vi "Helper SubVI - TDR Signal Simulation.vi"(6 "test parameters":T2={"Sample Rate [Hz]"=1000000.0, "Max Thickness [m]"=1.0, "SNR [dB]"=20.0} {"SNR [dB]" format="%.2f"; "Max Thickness [m]" format="%.2f"; "Sample Rate [Hz]" format="%.2p"}, 9 "target parameters":T1={"Reflectance"=0.0, "Phase Shift [Deg]"=-63.20559286450312} {"Reflectance" format="%.2f"}, 10 "path parameters":T3={"Thickness [m]"=0.43125, "Attenuation [dB/m]"=20.0, "Sonic Speed [m/s]"=1500.0} {"Sonic Speed [m/s]" format="%.2p"; "Attenuation [dB/m]" format="%.2f"; "Thickness [m]" format="%.4f"}, 11 "source chirplet":T4={"F Central [Hz]"=50000.0, "Bandwidth [Hz]"=50000.0, "Chirplet Length [m]"=0.2, "Amplitude [EU]"=10.0} {"Amplitude [EU]" format="%.2f"; "F Central [Hz]" format="%.2p"; "Bandwidth [Hz]" format="%.2p"; "Chirplet Length [m]" format="%.4f"}) -> (1 "noise":dbl=0.01 format="%.0p", 2 "incident chirplet":T5={"alpha"=0.00275625, "t0"=133.33333333333334, "omega"=0.314, "beta"=0.004710000000000001} {"beta" step=0.0001 format="%.2e"; "omega" format="%.2e"; "t0" format="%.3e"; "alpha" format="%.2e"}, 3 "time waveform":waveform(dbl), 4 "thickness between 2 samples":dbl format="%.2e")   [LabVIEW 2023]
doc: "Simulates a Time Domain Reflectometry (TDR) signal, which contains both the transmitted and the reflected chirplets."
uses:
  <vilib>/Analysis/NI_AALBase.lvlib
panel:
  out "length [sample]":i32=1600
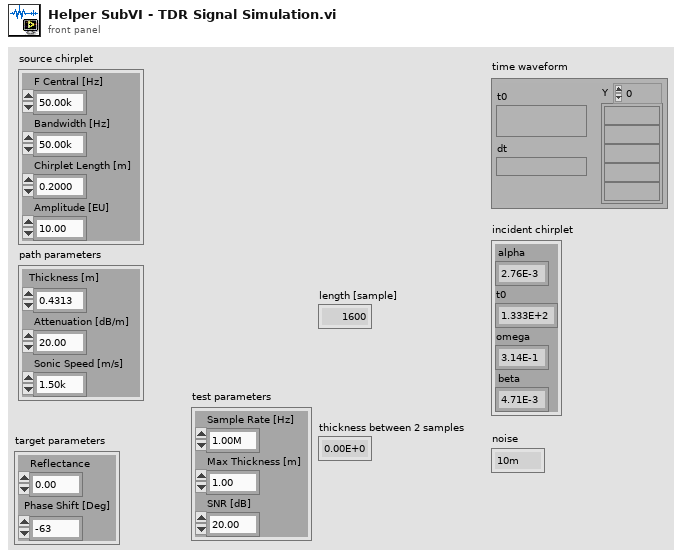
[diagram p1: front panel]
types:
  T1 = cluster{"Reflectance":dbl, "Phase Shift [Deg]":dbl}
  T2 = cluster{"Sample Rate [Hz]":dbl, "Max Thickness [m]":dbl, "SNR [dB]":dbl}
  T3 = cluster{"Thickness [m]":dbl, "Attenuation [dB/m]":dbl, "Sonic Speed [m/s]":dbl}
  T4 = cluster{"F Central [Hz]":dbl, "Bandwidth [Hz]":dbl, "Chirplet Length [m]":dbl, "Amplitude [EU]":dbl}
  T5 = cluster{"alpha":dbl, "t0":dbl, "omega":dbl, "beta":dbl}
  T6 = cluster{"F Central [Hz]":dbl, "Bandwidth [Hz]":dbl, "Chirplet Length [m]":dbl}
  T7 = cluster{"Sample Rate [Hz]":dbl, "Sonic Speed [m/s]":dbl}
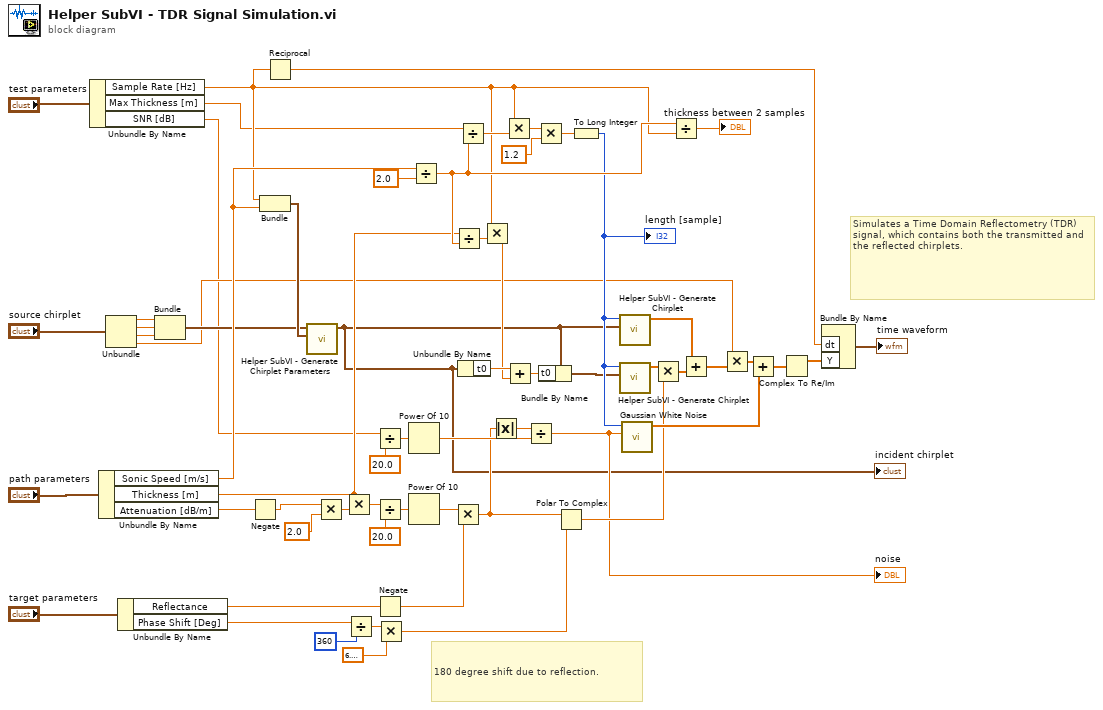
[diagram p0: block diagram]
diagram:
  # "Simulates a Time Domain Reflectometry (TDR) signal, which contains both the transmitted and the reflected chirplets."
  # "180 degree shift due to reflection."
  n1 = Unbundle By Name("test parameters") -> ("Sample Rate [Hz]"=w28:dbl, "Max Thickness [m]"=w27:dbl, "SNR [dB]"=w13:dbl)
  n2 = Unbundle By Name("path parameters") -> ("Sonic Speed [m/s]"=w30:dbl, "Thickness [m]"=w31:dbl, "Attenuation [dB/m]"=w32:dbl)
  n3 = Unbundle("source chirplet") -> ("F Central [Hz]"=w25:dbl, "Bandwidth [Hz]"=w24:dbl, "Chirplet Length [m]"=w23:dbl, "Amplitude [EU]"=w21:dbl)
  n4 = Unbundle By Name("target parameters") -> ("Reflectance"=w18:dbl, "Phase Shift [Deg]"=w19:dbl)
  n5 = Bundle("F Central [Hz]"=w25, "Bandwidth [Hz]"=w24, "Chirplet Length [m]"=w23) -> (w22:T6)  [unwired: 1 out]
  n6 = Negate(x=w32) -> (-x=w4:dbl)
  n7 = Bundle("Sample Rate [Hz]"=w28, "Sonic Speed [m/s]"=w30) -> (w36:T7)  [unwired: 1 out]
  n8 = Reciprocal(x=w28) -> (1/x=w8:dbl)
  n9 = call "Helper SubVI - Generate Chirplet Parameters.vi"("test conditions"=w36, "chirplet settings"=w22) -> ("chirplet parameters"=w2:T5)  [unwired: 1 in, 8 out]
  "incident chirplet" <- w2
  n10 = Multiply(x=w4, y=2.0) -> (x*y=w5:dbl)
  n11 = Multiply(x=w31, y=w5) -> (x*y=w51:dbl)
  n12 = Divide(x=w19, y=360) -> (x/y=w38:dbl)
  n13 = Divide(x=w13, y=20.0) -> (x/y=w12:dbl)
  n14 = Divide(x=w51, y=20.0) -> (x/y=w49:dbl)
  n15 = Negate ("180 degree shift due to reflection")(x=w18) -> (-x=w16:dbl)
  n16 = Multiply(x=w38, y=6.283185307179586 ("Pi Multiplied By 2")) -> (x*y=w15:dbl)
  n17 = Power Of 10(x=w12) -> (10^x=w11:dbl)
  n18 = Power Of 10(x=w49) -> (10^x=w47:dbl)
  n19 = Divide(x=w30, y=2.0) -> (x/y=w41:dbl)
  n20 = Multiply(x=w47, y=w16) -> (x*y=w10:dbl)
  n21 = Divide(x=w31, y=w41) -> (x/y=w55:dbl)
  n22 = Divide(x=w27, y=w41) -> (x/y=w56:dbl)
  n23 = Unbundle By Name(w2) -> ("t0"=w60:dbl)
  n24 = Multiply(x=w28, y=w55) -> (x*y=w54:dbl)
  n25 = Absolute Value(x=w10) -> (abs(x)=w6:dbl)
  n26 = Multiply(x=w28, y=w56) -> (x*y=w45:dbl)
  n27 = Add(x=w60, y=w54) -> (x+y=w59:dbl)
  n28 = Divide(x=w6, y=w11) -> (x/y=w7:dbl)
  "noise" <- w7
  n29 = Multiply(x=w45, y=1.2) -> (x*y=w46:dbl)
  n30 = Bundle By Name(cluster=w2, "t0"=w59) -> (w1:T5)
  n31 = Polar To Complex(1:w15, 2:w10) -> (0:w17:cdb)
  n32 = To Long Integer(number=w46) -> (32bit integer=w34:i32)
  "length [sample]" <- w34
  n33 = call "Helper SubVI - Generate Chirplet.vi"("parameter"=w2, "length"=w34) -> ("h(t)"=w58:cdb[])  [unwired: 1 in, 8 out]
  n34 = call "Helper SubVI - Generate Chirplet.vi"("parameter"=w1, "length"=w34) -> ("h(t)"=w48:cdb[])  [unwired: 1 in, 8 out]
  n35 = call <vilib>:"Gaussian White Noise.vi"("standard deviation"=w7, "samples"=w34) -> ("Gaussian noise pattern"=w43:dbl[])  [unwired: 8 in, 1 out]
  n36 = Multiply(x=w48, y=w17) -> (x*y=w57:cdb[])
  n37 = Divide(x=w41, y=w28) -> (x/y=→"thickness between 2 samples":dbl)
  n38 = Add(x=w58, y=w57) -> (x+y=w52:cdb[])
  n39 = Multiply(x=w21, y=w52) -> (x*y=w42:cdb[])
  n40 = Add(x=w42, y=w43) -> (x+y=w35:cdb[])
  n41 = Complex To Re/Im(x + iy=w35) -> (x=w61:dbl[])  [unwired: 1 out]
  n42 = Bundle By Name("dt"=w8, "Y"=w61) -> (→"time waveform":waveform(dbl))  [unwired: 1 out]
